vi "Build_Array_RGB.vi"(8 "error in (no error)":errorcluster caption="entrée d'erreur (pas d'erreur)", 11 "Load_SampleImage en entrée":refnum<class "Load_SampleImage.lvclass">) -> (0 "error out":errorcluster caption="sortie d'erreur", 2 "Image (RGB)":string[][](array[string]), 3 "Load_SampleImage en entrée":refnum<class "Load_SampleImage.lvclass">)   [LabVIEW 2020, in "Load_SampleImage.lvclass"]
uses:
  Load_SampleImage.lvclass
  Load_SampleImage.lvclass/Load_SampleImage.ctl
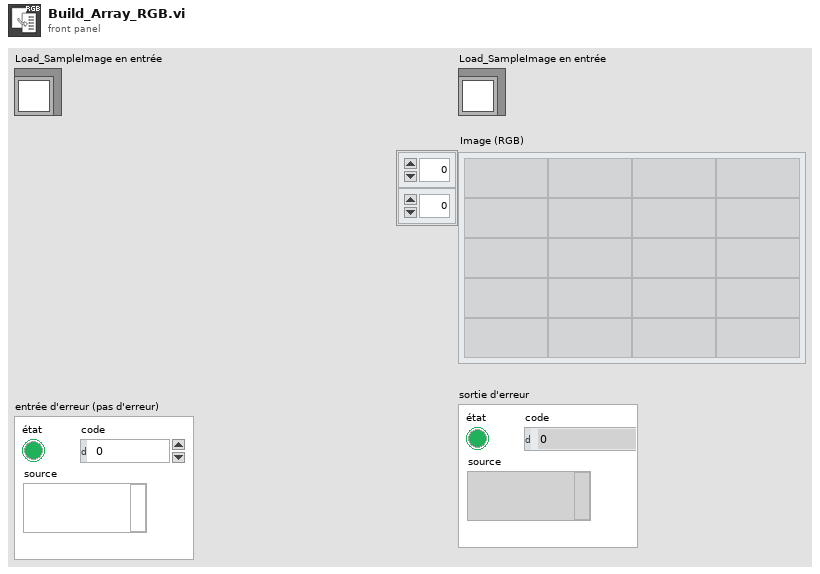
[diagram p1: front panel]
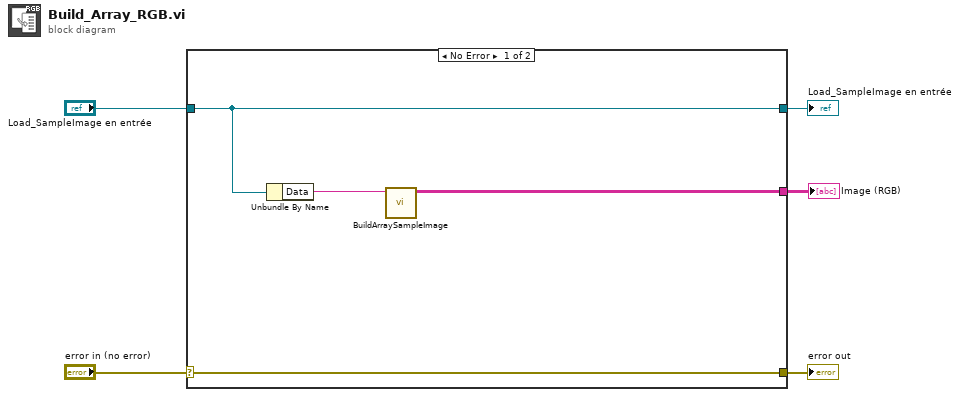
[diagram p0: block diagram]
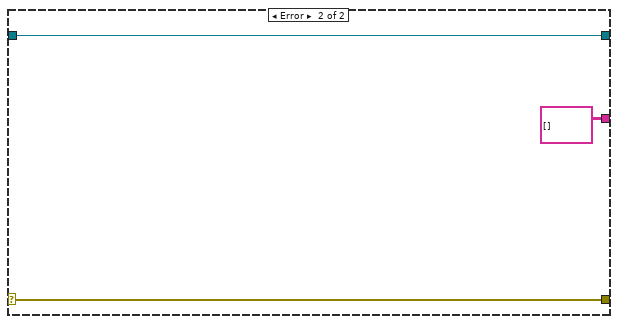
[diagram p2: hidden frame]
diagram:
  n1 = case shown="No Error" "error in (no error)" {
    selector: "error in (no error)" -> [w6 w12]
    tunnel: [w6 w12] -> w4
    tunnel: [w9 w11] -> w2
    tunnel: "Load_SampleImage en entrée" -> [w9 w11]
    tunnel: [w7 string[][] [] ("String 2DArray")] -> w1
    frame No Error {
      n2 = Unbundle By Name(w9) -> ("Data"=w8:string)
      n3 = call "BuildArraySampleImage.vi"("chaîne"=w8) -> ("Tableau"=w7:string[][])  [unwired: 10 in]
    }
    frame Error {
    }
  }
  "error out" <- w4
  "Load_SampleImage en entrée" <- w2
  "Image (RGB)" <- w1
